vi "P_I_D_INDIKATOR.vi"(4 "P I D":T2, 5 "Display?":enum16{"PID", "PI", "PD", "P", "I", "ID"}(ring), 6 "P I D 2":T2, 7 "P I D 6":T2, 8 "Array data":T1(array[cluster]), 9 "P I D 3":T2, 10 "P I D 4":T2, 11 "P I D 5":T2) -> (0 "Mean Array out":cluster{"History Data out":dbl[], dbl[]}, 3 "Cluster":T3={"P_POS"=1.0, "P_NEG"=1.0, "P_EXACT"=0.0, "I_POS"=1.0, "I_NEG"=1.0, "I_EXACT"=0.0, "D_POS"=1.0, "D_NEG"=1.0, "D_EXACT"=0.0} {"D_POS" scale=0.0..10.0; "I_POS" scale=0.0..10.0; "P_POS" scale=0.0..10.0})   [LabVIEW 2022 SP3]
uses:
  TypeDefs/P_I_D_Data_type.ctl
  <vilib>/Analysis/baseanly.llb/Mean (DBL).vi
  <vilib>/Analysis/NI_AALBase.lvlib
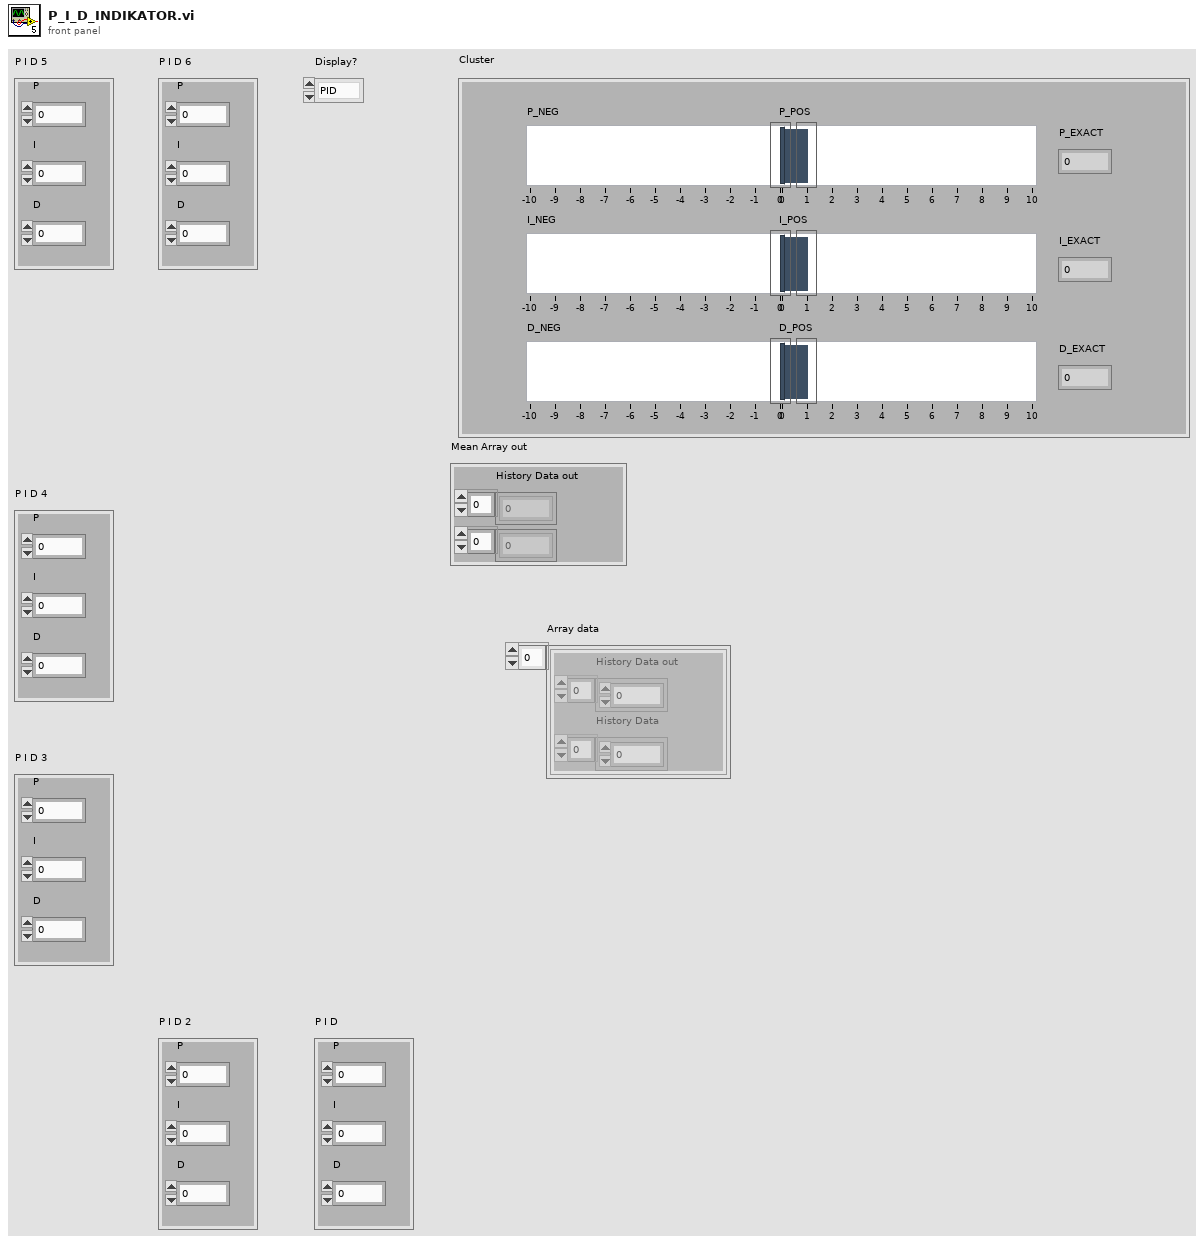
[diagram p1: front panel]
types:
  T1 = cluster{"History Data out":dbl[], "History Data":dbl[]}[]
  T2 = typedef "P_I_D_Data_type.ctl" = cluster{"P":dbl, "I":dbl, "D":dbl}
  T3 = cluster{"P_POS":dbl, "P_NEG":dbl, "P_EXACT":dbl, "I_POS":dbl, "I_NEG":dbl, "I_EXACT":dbl, "D_POS":dbl, "D_NEG":dbl, "D_EXACT":dbl}
  T4 = cluster{"History Data out":dbl[], "History Data":dbl[]}
  T5 = cluster{"P":dbl, "P":dbl, "P":dbl, "I":dbl, "I":dbl, "I":dbl, "D":dbl, "D":dbl, "D":dbl}
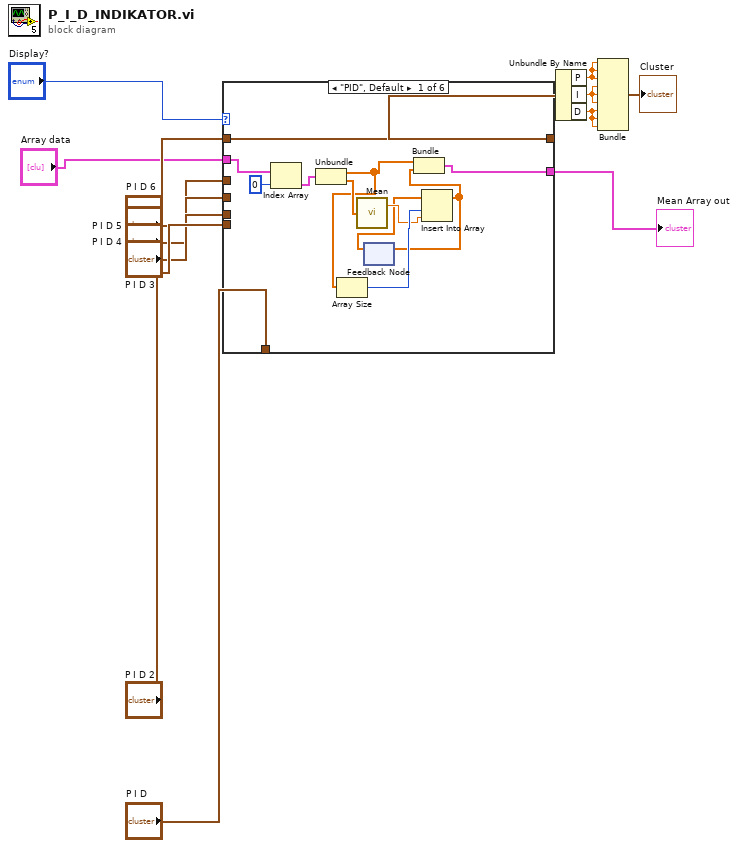
[diagram p0: block diagram]
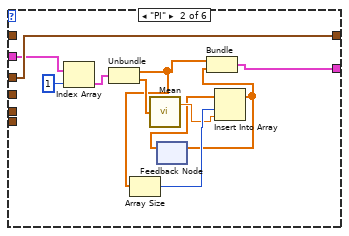
[diagram p2: hidden frame]
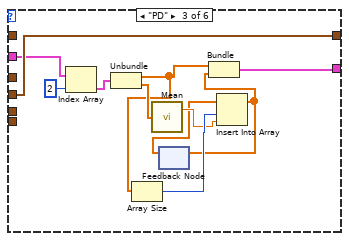
[diagram p3: hidden frame]
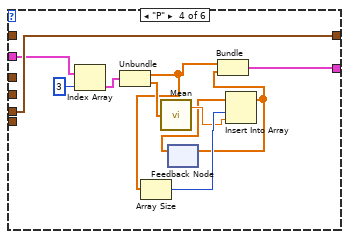
[diagram p4: hidden frame]
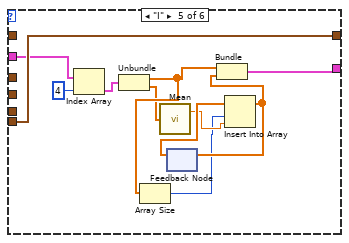
[diagram p5: hidden frame]
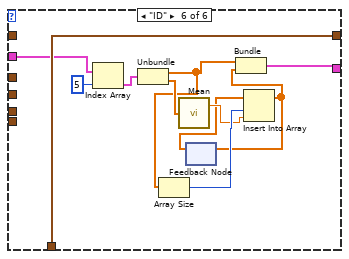
[diagram p6: hidden frame]
diagram:
  n1 = case shown="\"PID\", Default" "Display?" {
    tunnel: "P I D 6" -> [w25 _ _ _ _ _]
    tunnel: "P I D 5" -> [_ w36 _ _ _ _]
    tunnel: "P I D 4" -> [_ _ w47 _ _ _]
    tunnel: "P I D 3" -> [_ _ _ w58 _ _]
    tunnel: "P I D 2" -> [_ _ _ _ w69 _]
    tunnel: "P I D" -> [_ _ _ _ _ w80]
    tunnel: [w25 w36 w47 w58 w69 w80] -> w10
    tunnel: "Array data" -> [w24 w27 w38 w49 w60 w71]
    tunnel: [w15 w26 w37 w48 w59 w70] -> w1
    frame "PID", Default {
      n2 = Index Array(array=w24, index=0) -> (element=w22:T4)
      n3 = Unbundle(w22) -> ("History Data out"=w20:dbl[], "History Data"=w21:dbl[])
      n4 = Array Size(array=w20) -> (size(s)=w19:i32)
      n5 = call-poly <vilib>:"Mean.vi"("X"=w21) -> ("mean"=w18:dbl)  [unwired: 1 out]
      n6 = feedback #1() -> (w17:dbl[])  [unwired: 1 in]
      n7 = Insert Into Array(array=w17, index=w19, new element=w18) -> (w16:dbl[])
      n8 = feedback-in #1(w16) -> ()
      n9 = Bundle("History Data out"=w20, w16) -> (w15:cluster{"History Data out":dbl[], dbl[]})  [unwired: 1 in]
    }
    frame "PI" {
      n10 = Index Array(array=w27, index=1) -> (element=w34:T4)
      n11 = Unbundle(w34) -> ("History Data out"=w32:dbl[], "History Data"=w33:dbl[])
      n12 = Array Size(array=w32) -> (size(s)=w31:i32)
      n13 = call-poly <vilib>:"Mean.vi"("X"=w33) -> ("mean"=w30:dbl)  [unwired: 1 out]
      n14 = feedback #2() -> (w29:dbl[])  [unwired: 1 in]
      n15 = Insert Into Array(array=w29, index=w31, new element=w30) -> (w28:dbl[])
      n16 = feedback-in #2(w28) -> ()
      n17 = Bundle("History Data out"=w32, w28) -> (w26:cluster{"History Data out":dbl[], dbl[]})  [unwired: 1 in]
    }
    frame "PD" {
      n18 = Index Array(array=w38, index=2) -> (element=w45:T4)
      n19 = Unbundle(w45) -> ("History Data out"=w43:dbl[], "History Data"=w44:dbl[])
      n20 = Array Size(array=w43) -> (size(s)=w42:i32)
      n21 = call-poly <vilib>:"Mean.vi"("X"=w44) -> ("mean"=w41:dbl)  [unwired: 1 out]
      n22 = feedback #3() -> (w40:dbl[])  [unwired: 1 in]
      n23 = Insert Into Array(array=w40, index=w42, new element=w41) -> (w39:dbl[])
      n24 = feedback-in #3(w39) -> ()
      n25 = Bundle("History Data out"=w43, w39) -> (w37:cluster{"History Data out":dbl[], dbl[]})  [unwired: 1 in]
    }
    frame "P" {
      n26 = Index Array(array=w49, index=3) -> (element=w56:T4)
      n27 = Unbundle(w56) -> ("History Data out"=w54:dbl[], "History Data"=w55:dbl[])
      n28 = Array Size(array=w54) -> (size(s)=w53:i32)
      n29 = call-poly <vilib>:"Mean.vi"("X"=w55) -> ("mean"=w52:dbl)  [unwired: 1 out]
      n30 = feedback #4() -> (w51:dbl[])  [unwired: 1 in]
      n31 = Insert Into Array(array=w51, index=w53, new element=w52) -> (w50:dbl[])
      n32 = feedback-in #4(w50) -> ()
      n33 = Bundle("History Data out"=w54, w50) -> (w48:cluster{"History Data out":dbl[], dbl[]})  [unwired: 1 in]
    }
    frame "I" {
      n34 = Index Array(array=w60, index=4) -> (element=w62:T4)
      n35 = Unbundle(w62) -> ("History Data out"=w64:dbl[], "History Data"=w63:dbl[])
      n36 = Array Size(array=w64) -> (size(s)=w65:i32)
      n37 = call-poly <vilib>:"Mean.vi"("X"=w63) -> ("mean"=w66:dbl)  [unwired: 1 out]
      n38 = feedback #5() -> (w67:dbl[])  [unwired: 1 in]
      n39 = Insert Into Array(array=w67, index=w65, new element=w66) -> (w68:dbl[])
      n40 = feedback-in #5(w68) -> ()
      n41 = Bundle("History Data out"=w64, w68) -> (w59:cluster{"History Data out":dbl[], dbl[]})  [unwired: 1 in]
    }
    frame "ID" {
      n42 = Index Array(array=w71, index=5) -> (element=w78:T4)
      n43 = Unbundle(w78) -> ("History Data out"=w76:dbl[], "History Data"=w77:dbl[])
      n44 = Array Size(array=w76) -> (size(s)=w75:i32)
      n45 = call-poly <vilib>:"Mean.vi"("X"=w77) -> ("mean"=w74:dbl)  [unwired: 1 out]
      n46 = feedback #6() -> (w73:dbl[])  [unwired: 1 in]
      n47 = Insert Into Array(array=w73, index=w75, new element=w74) -> (w72:dbl[])
      n48 = feedback-in #6(w72) -> ()
      n49 = Bundle("History Data out"=w76, w72) -> (w70:cluster{"History Data out":dbl[], dbl[]})  [unwired: 1 in]
    }
  }
  "Mean Array out" <- w1
  n50 = Unbundle By Name(w10) -> ("P"=w11:dbl, "I"=w12:dbl, "D"=w13:dbl)
  n51 = Bundle("P"=w11, "P"=w11, "P"=w11, "I"=w12, "I"=w12, "I"=w12, "D"=w13, "D"=w13, "D"=w13) -> (→"Cluster":T5)  [unwired: 1 in]
